vi "Read Status.vi"(8 "error in (no error)":errorcluster, 11 "ExtFlatShutt in":refnum<class "ExtFlatShutt.lvclass">) -> (0 "error out":errorcluster, 2 "Status":bool, 3 "ExtFlatShutt out":refnum<class "ExtFlatShutt.lvclass">)   [LabVIEW 2016, in "ExtFlatShutt.lvclass"]
uses:
  ExtFlatShutt.lvclass
  Shutter.lvclass
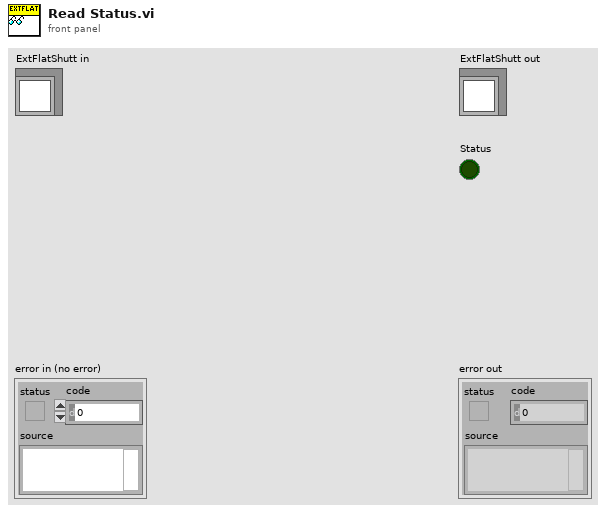
[diagram p1: front panel]
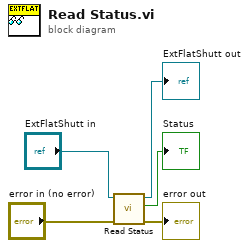
[diagram p0: block diagram]
diagram:
  n1 = call-parent "Read Status.vi"("error in (no error)"="error in (no error)", "Shutter in"="ExtFlatShutt in") -> ("error out"=→"error out":errorcluster, "Status"=→"Status":bool, "Shutter out"=→"ExtFlatShutt out":refnum<class "ExtFlatShutt.lvclass">)  [unwired: 7 in]
